vi "基础14.vi"() -> ()   [LabVIEW 2014]
panel:
  out "簇":cluster{"布尔":bool, "字符串":string}
  in  "报警":dbl(slide) scale=0.0..100.0
  out "温度计":dbl(slide) scale=0.0..100.0
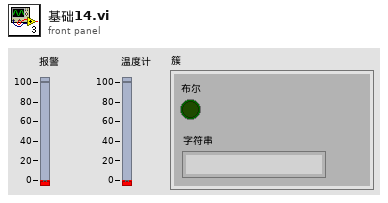
[diagram p1: front panel]
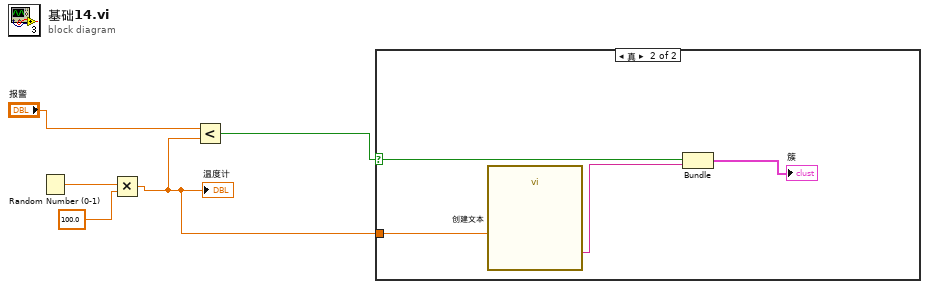
[diagram p0: block diagram]
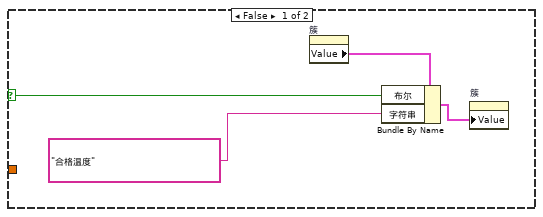
[diagram p2: hidden frame]
diagram:
  n1 = Random Number (0-1)() -> (number: 0 to 1=w5:dbl)
  n2 = Multiply(x=w5, y=100.0) -> (x*y=w1:dbl)
  "温度计" <- w1
  n3 = Less?(x="报警", y=w1) -> (x < y?=w2:bool)
  n4 = case shown="真" w2 {
    selector: w2 -> [w8 w10]
    tunnel: w1 -> [_ w12]
    frame False {
      n5 = property on="簇" class="Clust (严格)"() -> ("Value"=w9:cluster{"布尔":bool, "字符串":string})  [unwired: 2 in, 2 out]
      n6 = Bundle By Name(cluster=w9, "布尔"=w8, "字符串"="合格温度") -> (w6:cluster{"布尔":bool, "字符串":string})
      n7 = property on="簇" class="Clust (严格)"("Value"=w6) -> ()  [unwired: 2 in, 2 out]
    }
    frame True {
      n8 = call "创建文本"("n"=w12) -> ("Result"=w11:string)  [unwired: 13 in, 1 out]
      n9 = Bundle(w10, "Result"=w11) -> (→"簇":cluster{bool, "Result":string})  [unwired: 1 in]
    }
  }
